vi "Chaser.vi"   [LabVIEW 2015]
uses:
  <vilib>/Aledyne-TSXperts/Arduino Compatible Compiler for LabVIEW/Arduino Compatible Compiler for LabVIEW.lvlib
  <vilib>/Aledyne-TSXperts/Arduino Compatible Compiler for LabVIEW/Code Generator/Arduino APIs/RGB LED Strip/RGB Strip Mode.ctl
types:
  T1 = typedef "Arduino Compatible Compiler for LabVIEW.lvlib/RGB Strip Mode.ctl" = u16
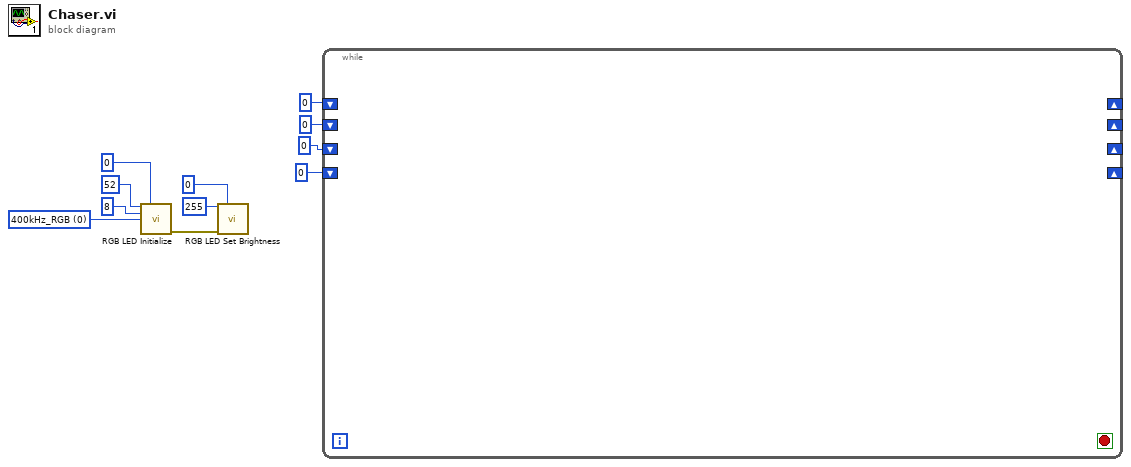
[diagram p0: block diagram]
diagram:
  w9 = T1 0 items=["400kHz_RGB"=0, "400kHz_GRB"=1, "400kHz_BRG"=4, "800kHz_RGB"=2, "800kHz_GRB"=3, "400kHz_BRG"=6] ("Mode")
  n1 = call <vilib>:"RGB LED Initialize.vi"("Number of Pixels"=u16 52, "Instance"=u8 0, "Pin"=u8 8, "Mode"=w9) -> ("error out"=w8:errorcluster)  [unwired: 11 in]
  n2 = call <vilib>:"RGB LED Set Brightness.vi"("Brightness"=u8 255, "Instance"=u8 0, "error in (no error)"=w8) -> ()  [unwired: 12 in, 1 out]
  n3 = while {
    shift-right: _ -> [_]
    shift-left: 0 -> [_]
    shift-right: _ -> [_]
    shift-left: 0 -> [_]
    shift-right: _ -> [_]
    shift-left: 0 -> [_]
    shift-right: _ -> [_]
    shift-left: 0 -> [_]
    stop <- _ stop-if-true
  }
